vi "cluster4image.vi"(11 "MaxProj 4":u16[][][](array[numeric])) -> (3 "Array":T1(array[cluster]))   [LabVIEW 2015]
panel:
  out "size(s) 2":i32
  out "size(s)":i32[](array[numeric])
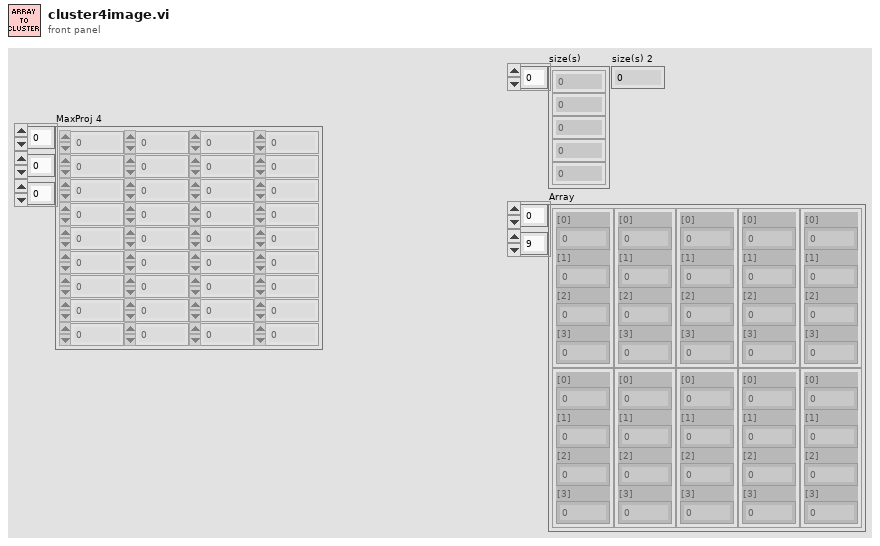
[diagram p1: front panel]
types:
  T1 = cluster{"[0]":u16, "[1]":u16, "[2]":u16, "[3]":u16}[][]
  T2 = cluster{"[0]":u16, "[1]":u16, "[2]":u16, "[3]":u16}
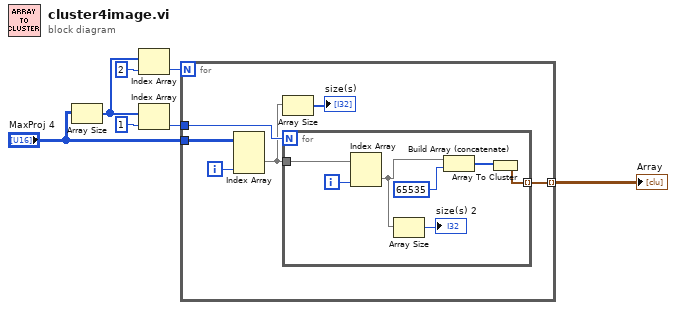
[diagram p0: block diagram]
diagram:
  n1 = Array Size(array="MaxProj 4") -> (size(s)=w2:i32[])
  n2 = Index Array(array=w2, index=2) -> (element=w4:i32)
  n3 = Index Array(array=w2, index=1) -> (element=w1:i32)
  n4 = for {
    N: w4 -> [_]
    tunnel: "MaxProj 4" -> [w10]
    tunnel: [w13] -> w7 mode=indexing
    tunnel: w1 -> [w11]
    i -> [w9]
    n5 = Index Array(array=w10, index (dim 2)=w9) -> (element=w8:u16[][])  [unwired: 2 in]
    n6 = Array Size(array=w8) -> (size(s)=→"size(s)":i32[])
    n7 = for {
      N: w11 -> [_]
      tunnel: [w14] -> w13 mode=indexing
      tunnel: w8 -> [w19]
      i -> [w18]
      n8 = Index Array(array=w19, index (col)=w18) -> (element=w17:u16[])  [unwired: 1 in]
      n9 = Array Size(array=w17) -> (size(s)=→"size(s) 2":i32)
      n10 = Build Array (concatenate)(w17, u16 65535 ("n")) -> (w15:u16[])
      n11 = Array To Cluster(array=w15) -> (cluster=w14:T2)
    }
  }
  "Array" <- w7
